vi "Read Output.vi"(8 "error in":errorcluster, 11 "N5745A in":refnum<class "5745A.lvclass">) -> (0 "error out":errorcluster, 2 "Output":bool, 3 "N5745A out":refnum<class "5745A.lvclass">)   [LabVIEW 2018, in "5745A.lvlib" / "5745A.lvclass"]
doc: "This Override method verifies if the N5745A instrument ouput is ON or OFF."
uses:
  5745A.lvclass
  builds/Power_Supply.lvlibp/Power Supply.lvclass
  C:/Users/Ron.Dexter.LUMINARTECH/Desktop/builds/Power_Supply.lvlibp/Power Supply.lvclass
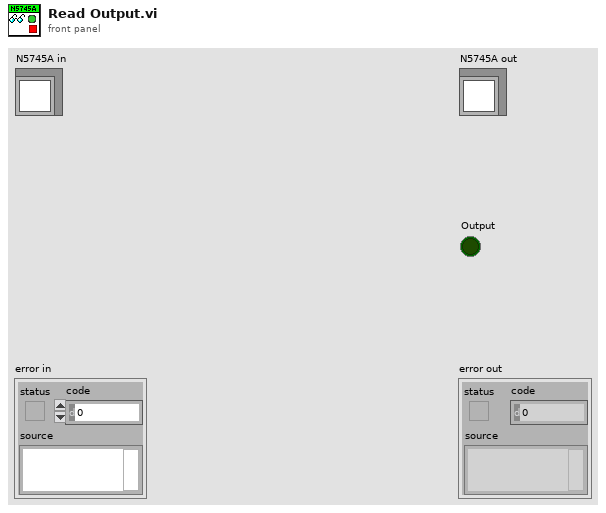
[diagram p1: front panel]
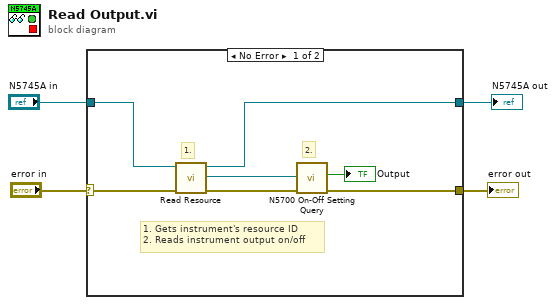
[diagram p0: block diagram]
diagram:
  n1 = case shown="No Error" "error in" {
    selector: "error in" -> [w10 w12]
    tunnel: "N5745A in" -> [w6 w13]
    tunnel: [w7 w12] -> w3
    tunnel: [w5 w13] -> w1
    frame No Error {
      # "1. Gets instrument's resource ID\n2. Reads instrument output on/off"
      # "2."
      # "1."
      n2 = call "Read Resource.vi"("error in"=w10, "Power Supply in"=w6) -> ("error out"=w8:errorcluster, "Resource"=w9:refnum<visa-resource-name>, "Power Supply out"=w5:refnum<class "5745A.lvclass">)  [unwired: 7 in]
      n3 = call <instrlib>:"N5700 On-Off Setting Query.vi"("error"=w8, "VISA"=w9) -> ("error out"=w7:errorcluster, "Output Set ON"=→"Output":bool)  [unwired: 5 in, 1 out]
    }
    frame Error {
    }
  }
  "error out" <- w3
  "N5745A out" <- w1
